vi "DMM_Scan PRD 32V-16C Close.vi"(0 "Scan Resources Handles In":T1={"DMM Handle"="", "MUX Handle"="", "Relays Debounce Time (ms)"=5, "Close all Shunts?"=TRUE}, 11 "error in":errorcluster) -> (15 "error out":errorcluster)   [LabVIEW 2021, in "DMM_Scan PXI RLY Driver 32V-16C.lvlib"]
doc: "Disconnects all Multiplexer/Shunt Relays and closes the NI-DMM and NI-SWITCH Scan session specifed in Scan Resource Handle In and releases all resources."
uses:
  DMM_Scan PXI RLY Driver 32V-16C.lvlib
  Typedefs/Scan Resource Handles In.ctl
  DMM Mixed Measurements/DMM_Mixed Measurement.lvlib
  Static Digital Path Generation/Switch_Static Digital Path Generation.lvlib
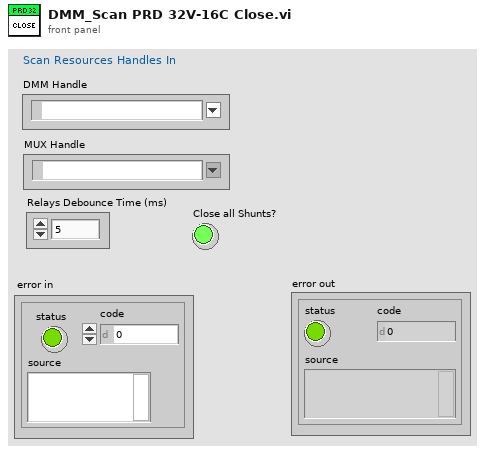
[diagram p1: front panel]
types:
  T1 = typedef "DMM_Scan PXI RLY Driver 32V-16C.lvlib/Scan Resource Handles In.ctl" = cluster{"DMM Handle":refnum<k15>, "MUX Handle":refnum<k15>, "Relays Debounce Time (ms)":u32, "Close all Shunts?":bool}
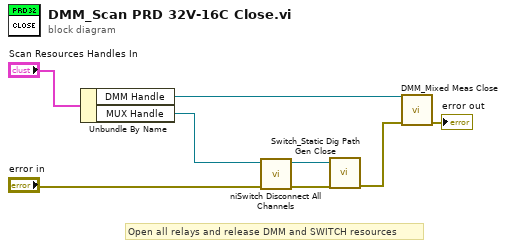
[diagram p0: block diagram]
diagram:
  # "Open all relays and release DMM and SWITCH resources"
  n1 = Unbundle By Name("Scan Resources Handles In") -> ("DMM Handle"=w6:refnum<k15>, "MUX Handle"=w2:refnum<k15>)
  n2 = call <instrlib>:"niSwitch Disconnect All Channels.vi"("error in (no error)"="error in", "instrument handle"=w2) -> ("error out"=w4:errorcluster, "instrument handle out"=w3:refnum<k15>)  [unwired: 8 in]
  n3 = call "Switch_Static Dig Path Gen Close.vi"("Switch Handle In"=w3, "error in"=w4) -> ("error out"=w7:errorcluster)  [unwired: 13 in]
  n4 = call "DMM_Mixed Meas Close.vi"("DMM Handle In"=w6, "error in"=w7) -> ("error out"=→"error out":errorcluster)  [unwired: 13 in]
